vi "loadSoftwareBinFinal.vi"() -> ()   [LabVIEW 2012]
uses:
  <vilib>/addons/database/Auxilliary.llb/DB Tools Cursor Type.ctl
  <vilib>/addons/database/Connection.llb/DB Tools Open Connec (Path).vi
  <vilib>/addons/database/Connection.llb/Conn Execute.vi
  <vilib>/addons/database/Recordset.llb/Rec Fetch Recordset Data (R).vi
  <vilib>/addons/database/Recordset.llb/Rec Destroy - Connection.vi
  <vilib>/addons/database/_DB Variant To Data/Database Variant To Data.xnode
  <vilib>/addons/database/NI_Database_API.lvlib
panel:
  out "recordset data":variant[][](array[variant])
  out "data":string
  out "error out":errorcluster
  out "concatenated string":string
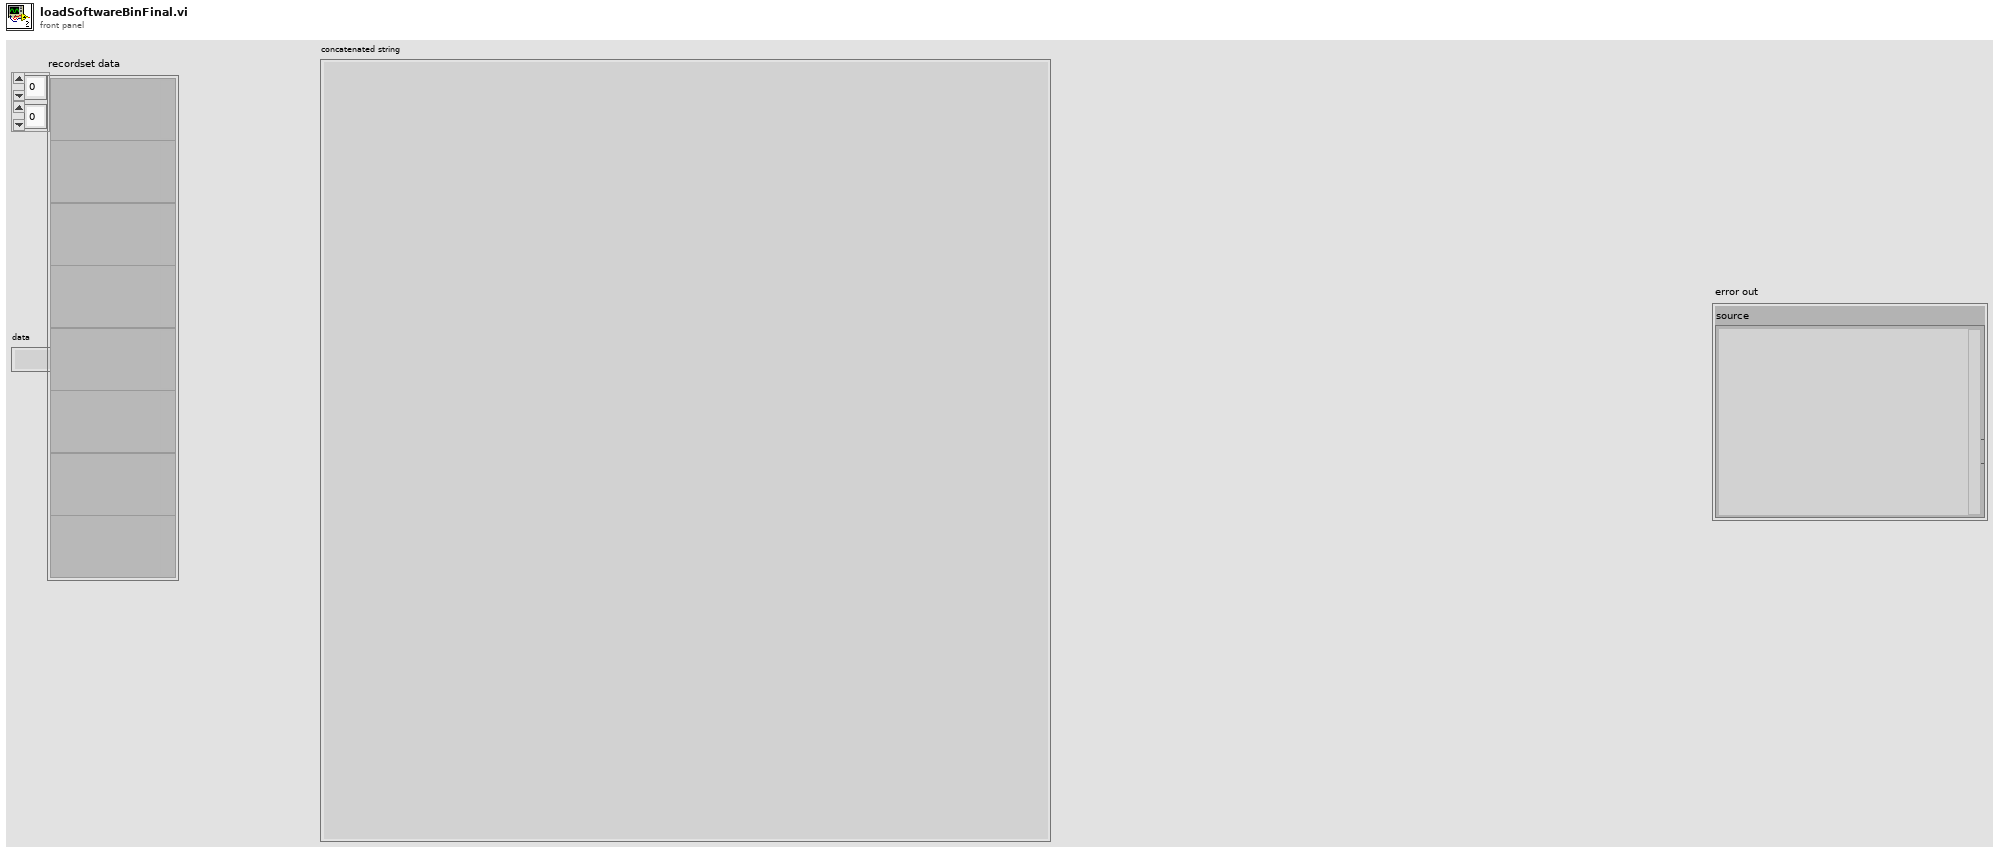
[diagram p1: front panel]
types:
  T1 = typedef "NI_Database_API.lvlib/DB Tools Cursor Type.ctl" = enum16{"forward-only", "keyset", "dynamic", "static"}
  T2 = typedef "NI_Database_API.lvlib/Conn ObjectReference.ctl" = refnum<k1>
  T3 = typedef "NI_Database_API.lvlib/Rec ObjectReference.ctl" = refnum<k1>
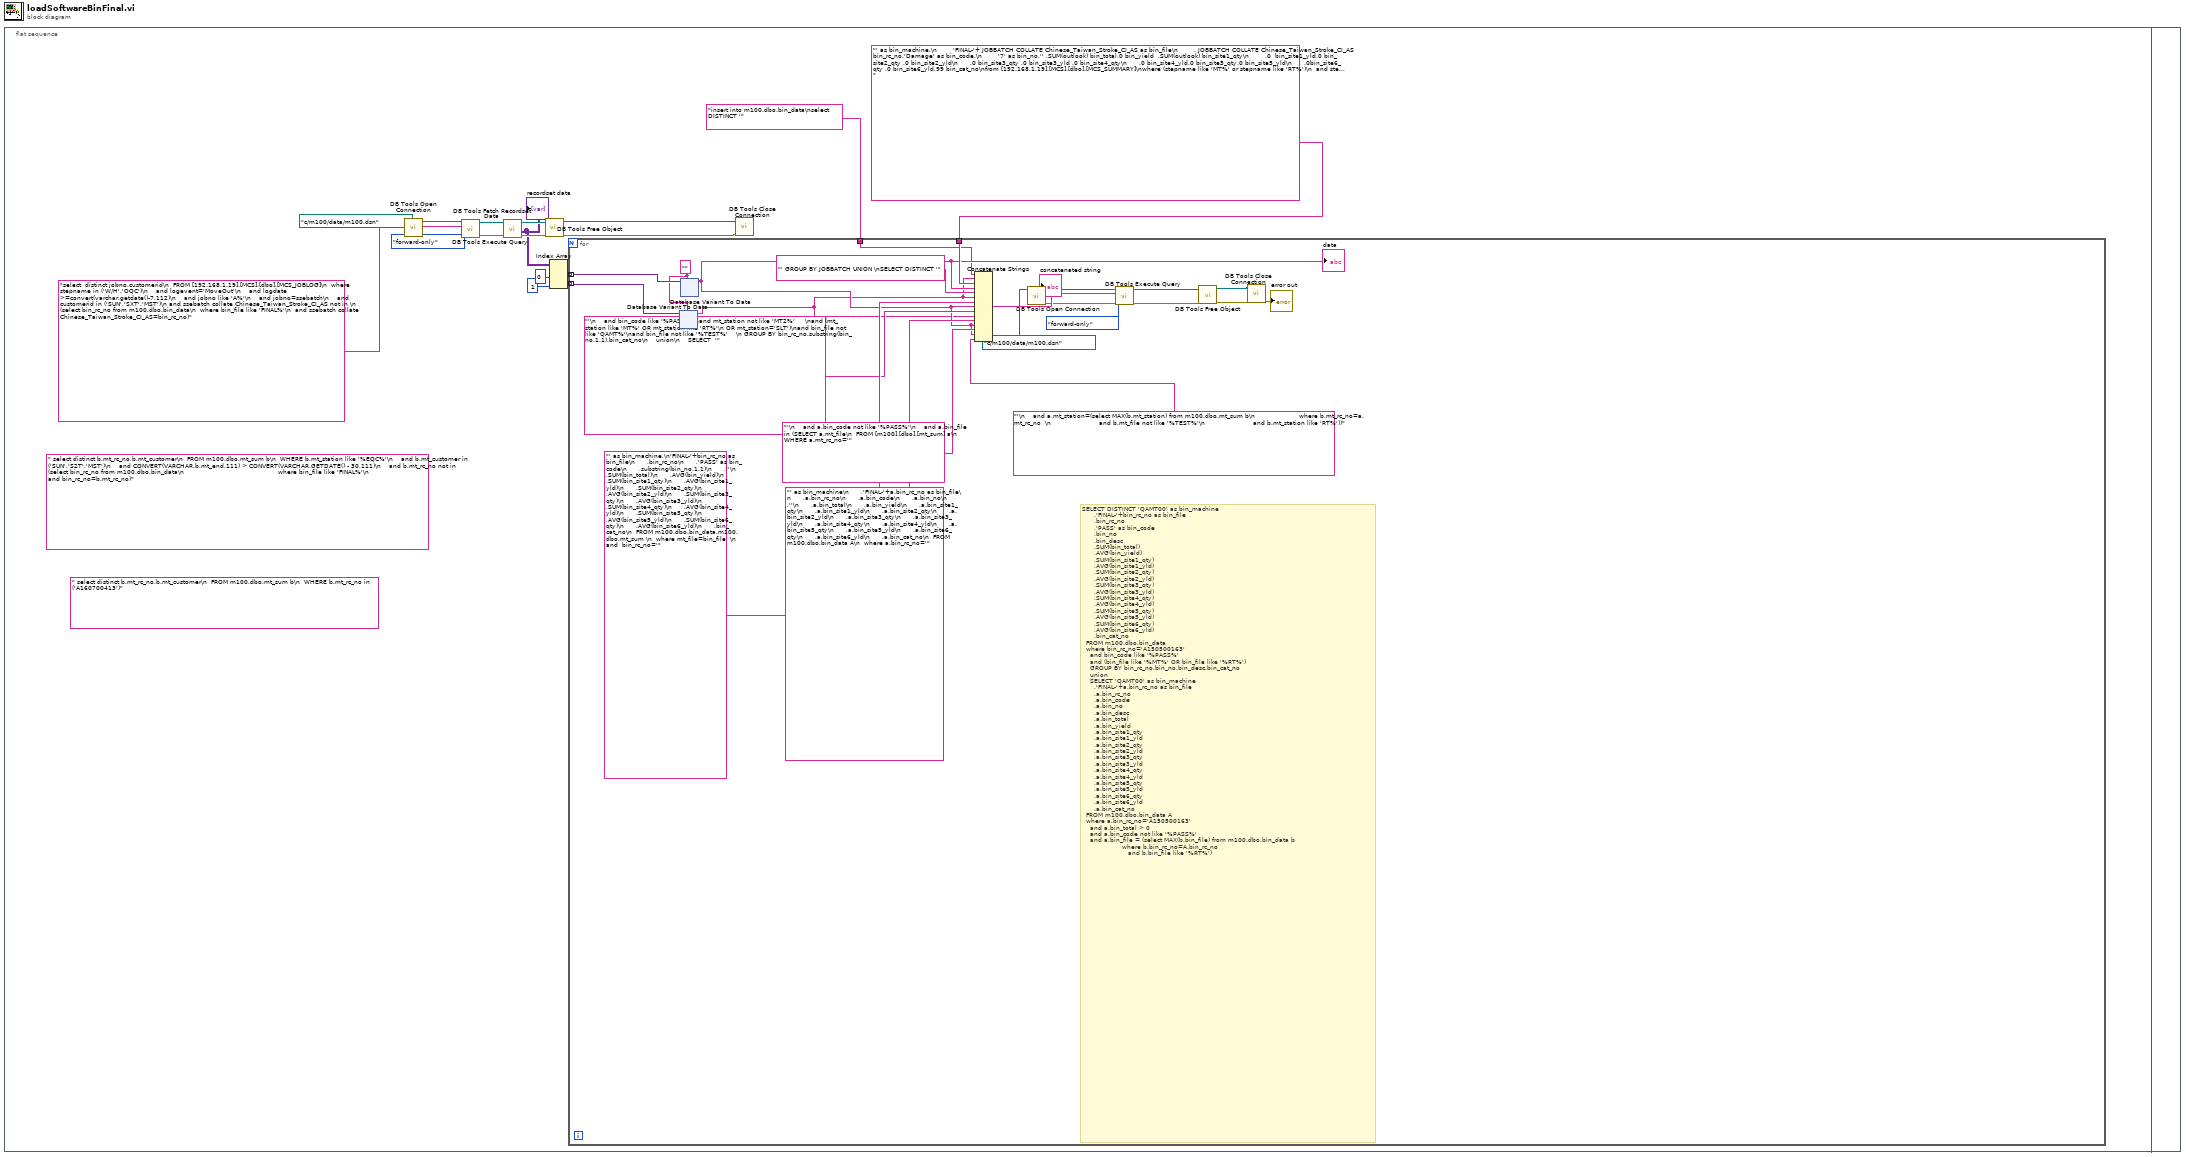
[diagram p0: block diagram]
diagram:
  n1 = flat-sequence {
    frame #0 {
      (unwired) " select distinct b.mt_rc_no,b.mt_customer\n  FROM m100.dbo.mt_sum b\n  WHERE b.mt_rc_no in ('A160700413')" ("SQL query")
      (unwired) " select distinct b.mt_rc_no,b.mt_customer\n  FROM m100.dbo.mt_sum b\n  WHERE b.mt_station like '%EQC%'\n    and b.mt_customer in ('SUN','S2T','MST')\n    and CONVERT(VARCHAR,b.mt_end,111) > CONVERT(VARCHAR,GETDATE() - 30,111)\n    and b.mt_rc_no not in (select bin_rc_no from m100.dbo.bin_data\n                                               where bin_file like 'FINAL%'\n                                                    and bin_rc_no=b.mt_rc_no)" ("SQL query")
      n2 = call-poly <vilib>:"DB Tools Open Connection.vi"("connection information"=path "c:/m100/data/m100.dsn") -> ("error out"=w15:errorcluster, "connection reference"=w18:T2)  [unwired: 7 in]
      n3 = call-poly <vilib>:"DB Tools Execute Query.vi"("error in (no error)"=w15, "cursor type"=DB_Tools_Cursor_Type."forward-only", "SQL query"="select  distinct jobno,customerid\n  FROM [192.168.1.19].[MCS].[dbo].[MCS_JOBLOG]\n  where  stepname in ('W/H','OQC')\n    and logevent='MoveOut'\n    and logdate >=convert(varchar,getdate()-7,112)\n    and jobno like 'A%'\n    and jobno=ssebatch\n    and customerid in ('SUN','SXT','MST')\n and ssebatch collate Chinese_Taiwan_Stroke_CI_AS not in \n (select bin_rc_no from m100.dbo.bin_data\n  where bin_file like 'FINAL%'\n  and ssebatch collate Chinese_Taiwan_Stroke_CI_AS=bin_rc_no)", "connection reference"=w18) -> ("error out"=w14:errorcluster, "recordset reference"=w17:T3)  [unwired: 4 in]
      n4 = call-poly <vilib>:"DB Tools Fetch Recordset Data.vi"("error in (no error)"=w14, "recordset reference"=w17) -> ("error out"=w13:errorcluster, "recordset data"=w10:variant[][], "recordset reference out"=w16:T3)  [unwired: 3 in]
      "recordset data" <- w10
      n5 = call-poly <vilib>:"DB Tools Free Object.vi"("error in (no error)"=w13, "recordset reference"=w16) -> ("error out"=w6:errorcluster, "connection reference"=w7:T2)  [unwired: 8 in]
      n6 = Index Array(array=w10, index (col) #1=0 ("disabled index (col)"), index (col) #2=1 ("index (col)")) -> (element #1=w8:variant[], element #2=w4:variant[])  [unwired: 2 in]
      n7 = for {
        tunnel: w8 -> [w41] mode=indexing
        tunnel: w4 -> [w29] mode=indexing
        tunnel: "' as bin_machine,\n        'FINAL-'+ JOBBATCH COLLATE Chinese_Taiwan_Stroke_CI_AS as bin_file\n        , JOBBATCH COLLATE Chinese_Taiwan_Stroke_CI_AS bin_rc_no,'Damage' as bin_code,\n        '7' as bin_no,'' ,SUM(outlook) bin_total,0 bin_yield  ,SUM(outlook) bin_site1_qty\n        ,0  bin_site1_yld,0 bin_site2_qty ,0 bin_site2_yld\n      ,0 bin_site3_qty ,0 bin_site3_yld ,0 bin_site4_qty\n      ,0 bin_site4_yld,0 bin_site5_qty,0 bin_site5_yld\n      ,0bin_site6_qty ,0 bin_site6_yld,99 bin_cat_no\nfrom [192.168.1.19].[MCS].[dbo].[MCS_SUMMARY]\nwhere (stepname like 'MT%' or stepname like 'RT%')\n  and stepname not like 'MT2%'\n  and outlook > 0\n  and JOBBATCH = '" -> [w22]
        tunnel: "insert into m100.dbo.bin_data\nselect DISTINCT '" -> [w20]
        w28 = ""
        # "SELECT DISTINCT 'QAMT00' as bin_machine\n      ,'FINAL-'+bin_rc_no as bin_file\n      ,bin_rc_no\n      ,'PASS' as bin_code\n      ,bin_no\n      ,bin_desc\n      ,SUM(bin_total)\n      ,AVG(bin_yield)\n      ,SUM(bin_site1_qty)\n      ,AVG(bin_site1_yld)\n      ,SUM(bin_site2_qty)\n      ,AVG(bin_site2_yld)\n      ,SUM(bin_site3_qty)\n      ,AVG(bin_site3_yld)\n      ,SUM(bin_site4_qty)\n      ,AVG(bin_site4_yld)\n      ,SUM(bin_site5_qty)\n      ,AVG(bin_site5_yld)\n      ,SUM(bin_site6_qty)\n      ,AVG(bin_site6_yld)\n      ,bin_cat_no\n  FROM m100.dbo.bin_data\n  where bin_rc_no='A150500163'\n    and bin_code like '%PASS%'\n    and (bin_file like '%MT%' OR bin_file like '%RT%')\n    GROUP BY bin_rc_no,bin_no,bin_desc,bin_cat_no\n    union\n    SELECT 'QAMT00' as bin_machine\n      ,'FINAL-'+a.bin_rc_no as bin_file\n      ,a.bin_rc_no\n      ,a.bin_code\n      ,a.bin_no\n      ,a.bin_desc\n      ,a.bin_total\n      ,a.bin_yield\n      ,a.bin_site1_qty\n      ,a.bin_site1_yld\n      ,a.bin_site2_qty\n      ,a.bin_site2_yld\n      ,a.bin_site3_qty\n      ,a.bin_site3_yld\n      ,a.bin_site4_qty\n      ,a.bin_site4_yld\n      ,a.bin_site5_qty\n      ,a.bin_site5_yld\n      ,a.bin_site6_qty\n      ,a.bin_site6_yld\n      ,a.bin_cat_no\n  FROM m100.dbo.bin_data A\n  where a.bin_rc_no='A150500163'\n    and a.bin_total > 0\n    and a.bin_code not like '%PASS%'\n    and a.bin_file = (select MAX(b.bin_file) from m100.dbo.bin_data b\n                    where b.bin_rc_no=A.bin_rc_no\n                       and b.bin_file like '%RT%')"
        n8 = xnode "Database Variant To Data"("database variant"=w29, "type"=w28) -> ("data"=w19:string)  [unwired: 1 in, 1 out]
        n9 = xnode "Database Variant To Data"("database variant"=w41, "type"=w28) -> ("data"=w21:string)  [unwired: 1 in, 1 out]
        "data" <- w21
        n10 = Concatenate Strings(w20, w19, w22, w21, "' GROUP BY JOBBATCH UNION \nSELECT DISTINCT '" ("string"), w19, "' as bin_machine,\n'FINAL-'+bin_rc_no as bin_file\n      ,bin_rc_no\n      ,'PASS' as bin_code\n      ,substring(bin_no,1,1)\n      ,''\n      ,SUM(bin_total)\n      ,AVG(bin_yield)\n      ,SUM(bin_site1_qty)\n      ,AVG(bin_site1_yld)\n      ,SUM(bin_site2_qty)\n      ,AVG(bin_site2_yld)\n      ,SUM(bin_site3_qty)\n      ,AVG(bin_site3_yld)\n      ,SUM(bin_site4_qty)\n      ,AVG(bin_site4_yld)\n      ,SUM(bin_site5_qty)\n      ,AVG(bin_site5_yld)\n      ,SUM(bin_site6_qty)\n      ,AVG(bin_site6_yld)\n      ,bin_cat_no\n  FROM m100.dbo.bin_data,m100.dbo.mt_sum \n  where mt_file=bin_file  \n  and  bin_rc_no='" ("string"), w21, "'\n    and bin_code like '%PASS%'\nand mt_station not like 'MT2%'     \nand (mt_station like 'MT%' OR mt_station like 'RT%'\n OR mt_station='SLT')\nand bin_file not like 'QAMT%'\nand bin_file not like '%TEST%'    \n GROUP BY bin_rc_no,substring(bin_no,1,1),bin_cat_no\n    union\n    SELECT  '" ("string"), w19, "' as bin_machine\n      ,'FINAL-'+a.bin_rc_no as bin_file\n      ,a.bin_rc_no\n      ,a.bin_code\n      ,a.bin_no\n      ,''\n      ,a.bin_total\n      ,a.bin_yield\n      ,a.bin_site1_qty\n      ,a.bin_site1_yld\n      ,a.bin_site2_qty\n      ,a.bin_site2_yld\n      ,a.bin_site3_qty\n      ,a.bin_site3_yld\n      ,a.bin_site4_qty\n      ,a.bin_site4_yld\n      ,a.bin_site5_qty\n      ,a.bin_site5_yld\n      ,a.bin_site6_qty\n      ,a.bin_site6_yld\n      ,a.bin_cat_no\n  FROM m100.dbo.bin_data A\n  where a.bin_rc_no='" ("string"), w21, "'\n    and a.bin_code not like '%PASS%'\n    and a.bin_file in (SELECT a.mt_file\n  FROM [m100].[dbo].[mt_sum] a\n  WHERE a.mt_rc_no='" ("string"), w21, "'\n    and a.mt_station=(select MAX(b.mt_station) from m100.dbo.mt_sum b\n                      where b.mt_rc_no=a.mt_rc_no  \n                        and b.mt_file not like '%TEST%'\n                        and b.mt_station like 'RT%'))" ("string")) -> (w39:string)
        "concatenated string" <- w39
        n11 = call-poly <vilib>:"DB Tools Open Connection.vi"("connection information"=path "c:/m100/data/m100.dsn") -> ("error out"=w37:errorcluster, "connection reference"=w38:T2)  [unwired: 7 in]
        n12 = call-poly <vilib>:"DB Tools Execute Query.vi"("error in (no error)"=w37, "cursor type"=DB_Tools_Cursor_Type."forward-only", "SQL query"=w39, "connection reference"=w38) -> ("error out"=w31:errorcluster, "recordset reference"=w30:T3)  [unwired: 4 in]
        n13 = call-poly <vilib>:"DB Tools Free Object.vi"("error in (no error)"=w31, "recordset reference"=w30) -> ("error out"=w34:errorcluster, "connection reference"=w35:T2)  [unwired: 8 in]
        n14 = call <vilib>:"DB Tools Close Connection.vi"("error in (no error)"=w34, "connection reference"=w35) -> ("error out"=→"error out":errorcluster)  [unwired: 5 in]
      }
      n15 = call <vilib>:"DB Tools Close Connection.vi"("error in (no error)"=w6, "connection reference"=w7) -> ()  [unwired: 5 in, 1 out]
    }
    frame #1 {
    }
  }
